vi "LOEM_Lvxy_Measurement.vi"() -> ()   [LabVIEW 2019]
uses:
  C:/Program Files (x86)/National Instruments/LabVIEW 2019/LC-MISDK.dll
  Program Files (x86)/National Instruments/LabVIEW 2019/LC-MISDK.dll
panel:
  out "Lv Display":dbl
  out "Lv 2":dbl
  out "error out":errorcluster
  in  "Calibration Ch":i32(ring) items=["U00", "U01", "U02", "U03", "U04"]
  in  "ManualMeasurementTime":dbl=0.1
  out "y":dbl
  out "x":dbl
  out "Lv":dbl
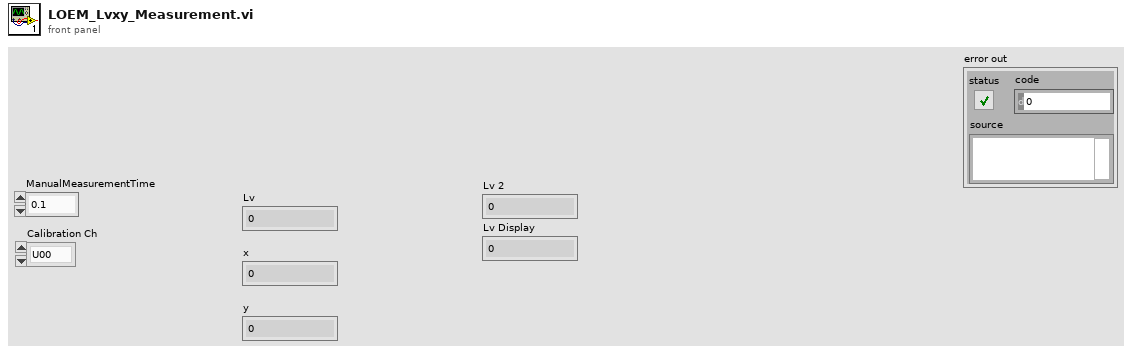
[diagram p1: front panel]
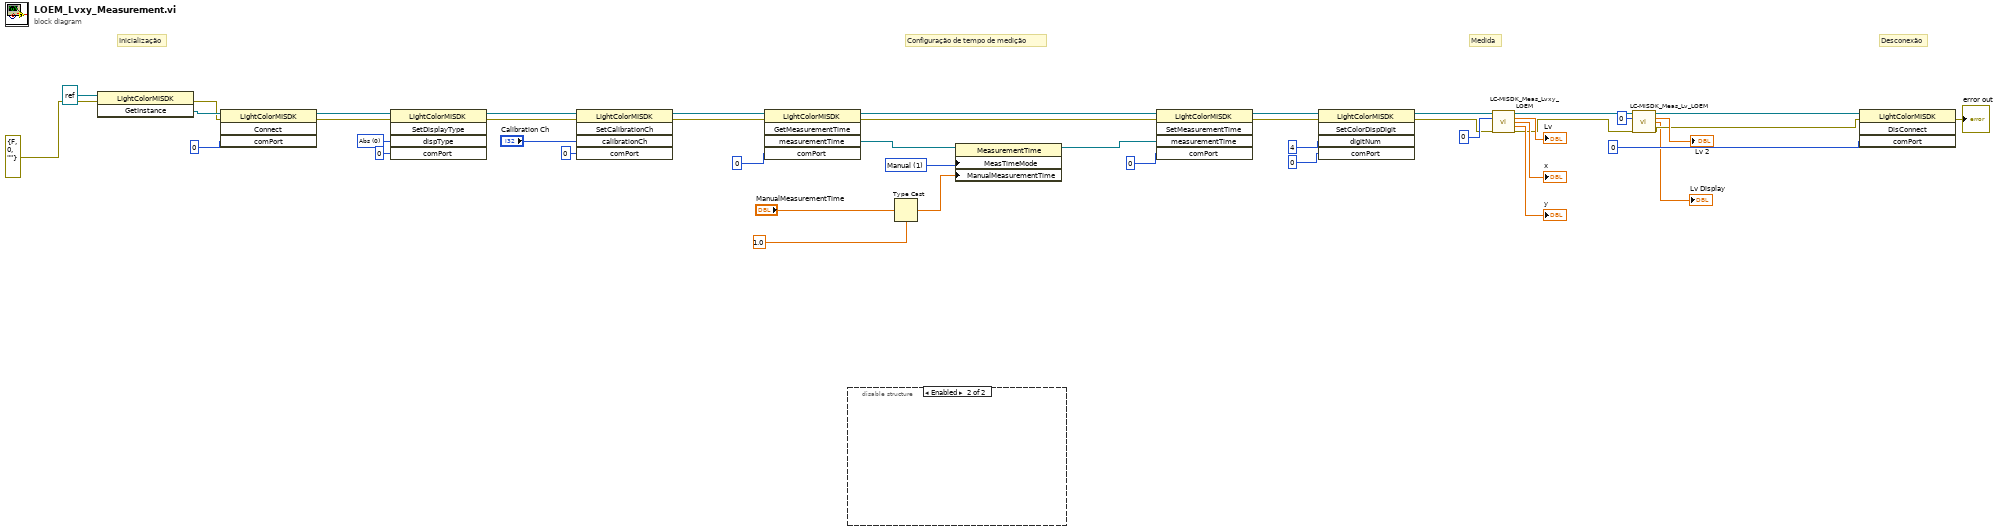
[diagram p0: block diagram]
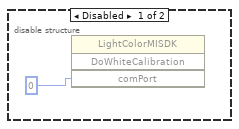
[diagram p2: hidden frame]
diagram:
  w21 = 0 items=["Abs", "Diff", "Ratio"] ("dispType")
  w37 = 1 items=["Auto", "Manual"] ("MeasTimeMode")
  # "Desconexão"
  # "Medida"
  # "Inicialização"
  # "Configuração de tempo de medição"
  n1 = invoke class="LightColorMISDK" method="GetInstance"(reference=refnum<k24> refnum, error in=errorcluster {"status"=FALSE, "code"=0, "source"=""} ("error in (no error)")) -> (error out=w15:errorcluster, "GetInstance"=w43:refnum<k24>)  [unwired: 1 in, 1 out]
  n2 = invoke class="LightColorMISDK" method="Connect"(reference=w43, error in=w15, "comPort"=0) -> (reference out=w23:refnum<k24>, error out=w14:errorcluster)  [unwired: 1 in, 2 out]
  n3 = invoke class="LightColorMISDK" method="SetDisplayType"(reference=w23, error in=w14, "dispType"=w21, "comPort"=0) -> (reference out=w20:refnum<k24>, error out=w13:errorcluster)  [unwired: 1 in, 3 out]
  n4 = invoke class="LightColorMISDK" method="SetCalibrationCh"(reference=w20, error in=w13, "calibrationCh"="Calibration Ch", "comPort"=0) -> (reference out=w19:refnum<k24>, error out=w12:errorcluster)  [unwired: 1 in, 3 out]
  n5 = invoke class="LightColorMISDK" method="GetMeasurementTime"(reference=w19, error in=w12, "comPort"=0) -> (reference out=w34:refnum<k24>, error out=w11:errorcluster, "measurementTime"=w33:refnum<k24>)  [unwired: 2 in, 2 out]
  n6 = disable-structure shown="Enabled" {
    frame Disabled {
      n7 = invoke class="LightColorMISDK" method="DoWhiteCalibration"("comPort"=0 ("DoWhiteCalibration")) -> ()  [unwired: 3 in, 4 out]
    }
    frame Enabled {
    }
  }
  n8 = Type Cast(type=1.0, x="ManualMeasurementTime") -> (*(type *) &x=w24:dbl)
  n9 = property class="MeasurementTime"(reference=w33, "MeasTimeMode"=w37, "ManualMeasurementTime"=w24) -> (reference out=w36:refnum<k24>)  [unwired: 1 in, 1 out]
  n10 = invoke class="LightColorMISDK" method="SetMeasurementTime"(reference=w34, error in=w11, "measurementTime"=w36, "comPort"=0) -> (reference out=w28:refnum<k24>, error out=w10:errorcluster)  [unwired: 1 in, 3 out]
  n11 = invoke class="LightColorMISDK" method="SetColorDispDigit"(reference=w28, error in=w10, "digitNum"=i16 4, "comPort"=0) -> (reference out=w27:refnum<k24>, error out=w9:errorcluster)  [unwired: 1 in, 3 out]
  n12 = call "LC-MISDK_Meas_Lvxy_LOEM.vi"(".NET reference"=w27, "comPort"=0, "error in"=w9) -> (".NET reference out"=w5:refnum<k24>, "Lv"=→"Lv":dbl, "x"=→"x":dbl, "y"=→"y":dbl, "error out"=w3:errorcluster)  [unwired: 7 in, 1 out]
  n13 = call "LC-MISDK_Meas_Lv_LOEM.vi"(".NET reference"=w5, "comPort"=0, "error in"=w3) -> (".NET reference out"=w4:refnum<k24>, "Lv"=→"Lv 2":dbl, "Lv Display"=→"Lv Display":dbl, "error out"=w2:errorcluster)  [unwired: 8 in, 1 out]
  n14 = invoke on="インボークノード" class="LightColorMISDK" method="DisConnect"(reference=w4, error in=w2, "comPort"=0) -> (error out=→"error out":errorcluster)  [unwired: 1 in, 3 out]
